vi "SVT STFT vs RPM (analog).vi"(0 "scaled signal [EU]":waveform(dbl), 1 "FFT block size":i32=1024 min=1, 2 "window":T3=1 items=["Rectangle"=0, "Hanning"=1, "Hamming"=2, "Blackman-Harris"=3, "Exact Blackman"=4, "Blackman"=5, "Flat Top"=6, "4 Term B-Harris "=7, "7 Term B-Harris"=8, "Low Sidelobe"=9, "Blackman Nuttall"=11, "Triangle"=30, "Bartlett-Hanning"=31, "Bohman"=32, "Parzen"=33, "Welch"=34, "Kaiser"=60, "Dolph-Chebyshev"=61, "Gaussian"=62], 5 "tach signal [V]":waveform(dbl), 7 "tach info":T2={"threshold [V]"=1.0, "pulse width (2)"=2, "avg on n pulses (2)"=2, "pulse/revolution (1)"=1} {"pulse/revolution (1)" min=1 step=1; "avg on n pulses (2)" min=2 step=1; "pulse width (2)" min=1; "threshold [V]" format="%.2f"}, 9 "rpm segment":T1={"from [rpm]"=2000.0, "to [rpm]"=4000.0, "rpm increment [rpm]"=100.0} {"rpm increment [rpm]" min=1.0 format="%.2f"; "to [rpm]" format="%.2f"; "from [rpm]" format="%.2f"}, 11 "error in (no error)":errorcluster, 12 "dB On (T)":bool=TRUE, 13 "weighting":u16(ring) items=["Linear", "A-weighting", "B-weighting", "C-weighting"]) -> (4 "power spectra [dB EU]":dbl[][](array[numeric]) format="%.2f", 6 "unit label":string, 8 "f0 and delta f [Hz]":cluster{"f0":dbl, "delta f":dbl} {"delta f" format="%.2f"; "f0" format="%.2f"}, 10 "rpm0 and delta rpm [rpm]":cluster{"rpm0":dbl, "delta rpm":dbl} {"delta rpm" format="%.2f"; "rpm0" format="%.2f"}, 14 "rpm vs. time":cluster{"time [s]":dbl[], "speed [rpm]":dbl[]} {"speed [rpm]" format="%.2f"; "time [s]" format="%.2f"}, 15 "error out":errorcluster)   [LabVIEW 2017]
doc: "Performs a short-time Fourier transform (STFT) on <B>scaled signal [EU]</B> as a function of the rotational speed recorded by <B>tach signal [V]</B> and returns the power spectrum at the specified rotational speeds."
uses:
  <vilib>/Analysis/4window.llb/windowTd.ctl
  <vilib>/Analysis/NI_AALPro.lvlib
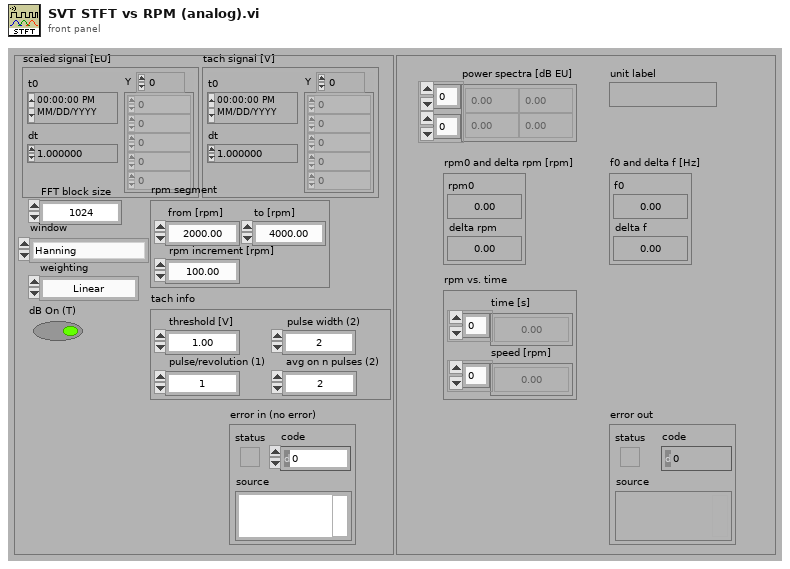
[diagram p1: front panel]
types:
  T1 = cluster{"from [rpm]":dbl, "to [rpm]":dbl, "rpm increment [rpm]":dbl}
  T2 = cluster{"threshold [V]":dbl, "pulse width (2)":i32, "avg on n pulses (2)":i32, "pulse/revolution (1)":i32}
  T3 = typedef "NI_AALPro.lvlib/windowTd.ctl" = u32
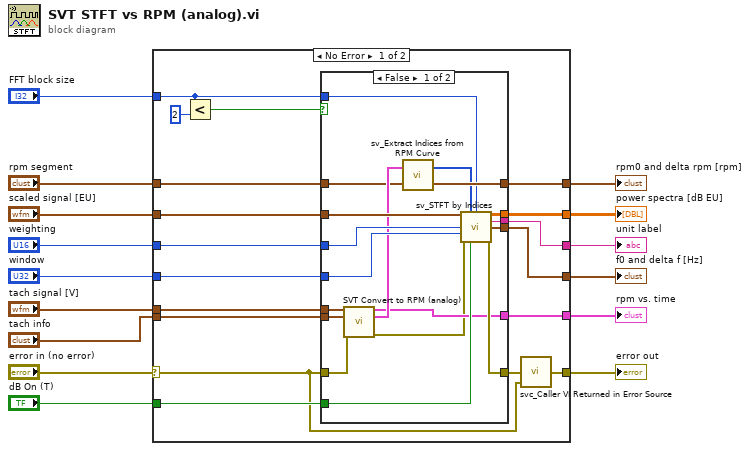
[diagram p0: block diagram]
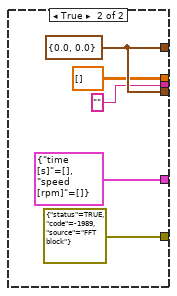
[diagram p2: hidden frame]
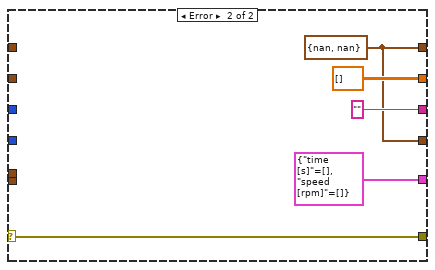
[diagram p3: hidden frame]
diagram:
  n1 = case shown="No Error" "error in (no error)" {
    selector: "error in (no error)" -> [w16 w61]
    tunnel: [w33 w57] -> w15
    tunnel: "FFT block size" -> [w20 _]
    tunnel: "dB On (T)" -> [w32 _]
    tunnel: "window" -> [w31 _]
    tunnel: [w30 dbl[][] [] ("power spectra [dB EU]")] -> w11
    tunnel: [w29 "" ("unit label")] -> w10
    tunnel: [w28 w57] -> w9
    tunnel: "rpm segment" -> [w18 _]
    tunnel: [w23 cluster{"time [s]":dbl[], "speed [rpm]":dbl[]} {"time [s]"=[], "speed [rpm]"=[]} ("rpm vs. time")] -> w7
    tunnel: "tach info" -> [w22 _]
    tunnel: "tach signal [V]" -> [w21 _]
    tunnel: "weighting" -> [w27 _]
    tunnel: "scaled signal [EU]" -> [w26 _]
    tunnel: [w24 w61] -> w2
    frame No Error {
      n2 = Less?(x=w20, y=2) -> (x < y?=w17:bool)
      n3 = case shown="False" w17 {
        tunnel: [w51 w55] -> w33
        tunnel: w32 -> [w50 _]
        tunnel: w31 -> [w49 _]
        tunnel: [w48 dbl[][] [] ("power spectra [dB EU]")] -> w30
        tunnel: [w47 "" ("unit label")] -> w29
        tunnel: [w46 w55] -> w28
        tunnel: w27 -> [w45 _]
        tunnel: w26 -> [w44 _]
        tunnel: [w43 errorcluster {"status"=TRUE, "code"=-1989, "source"="FFT block"} ("error out")] -> w25
        tunnel: [w41 cluster{"time [s]":dbl[], "speed [rpm]":dbl[]} {"time [s]"=[], "speed [rpm]"=[]} ("rpm vs. time")] -> w23
        tunnel: w22 -> [w40 _]
        tunnel: w21 -> [w39 _]
        tunnel: w16 -> [w38 _]
        tunnel: w20 -> [w35 _]
        tunnel: w18 -> [w34 _]
        frame False {
          n4 = call <vilib>:"SVT Convert to RPM (analog).vi"("tach signal [V]"=w39, "tach info"=w40, "error in (no error)"=w38) -> ("rpm vs. time"=w41:cluster{"time [s]":dbl[], "speed [rpm]":dbl[]}, "rpm vs. indices"=w42:cluster{"indices":dbl[], "speed [rpm]":dbl[]}, "error out"=w37:errorcluster)  [unwired: 10 in]
          n5 = call <vilib>:"sv_Extract Indices from RPM Curve.vi"("rpm segment"=w34, "rpm vs. indices"=w42) -> ("rpm0 and delta rpm [rpm]"=w51:cluster{"rpm0":dbl, "delta rpm":dbl}, "indices"=w36:i32[])
          n6 = call <vilib>:"sv_STFT by Indices.vi"("scaled signal [EU]"=w44, "indices"=w36, "FFT block size"=w35, "weighting"=w45, "window"=w49, "error in (no error)"=w37, "dB On (T)"=w50) -> ("power spectra [dB EU]"=w48:dbl[][], "unit label"=w47:string, "f0 and delta f [Hz]"=w46:cluster{"f0":dbl, "delta f":dbl}, "error out"=w43:errorcluster)  [unwired: 5 in]
        }
        frame True {
          w55 = cluster{"rpm0":dbl, "delta rpm":dbl} {"rpm0"=0.0, "delta rpm"=0.0} ("rpm0 and delta rpm [rpm]")
        }
      }
      n7 = call <vilib>:"svc_Caller VI Returned in Error Source.vi"("warning input to caller"=w16, "error in (no error)"=w25) -> ("error out"=w24:errorcluster)  [unwired: 3 in]
    }
    frame Error {
      w57 = cluster{"rpm0":dbl, "delta rpm":dbl} {"rpm0"=nan, "delta rpm"=nan} ("rpm0 and delta rpm [rpm]")
    }
  }
  "power spectra [dB EU]" <- w11
  "rpm0 and delta rpm [rpm]" <- w15
  "f0 and delta f [Hz]" <- w9
  "unit label" <- w10
  "rpm vs. time" <- w7
  "error out" <- w2
